vi "Convert TDMS to Excel.vi"(8 "error in":errorcluster, 9 "Show Configure Dialog?":bool, 10 "Remove Extra Properties? (T)":bool=TRUE, 11 "Path to TDMS/TDM File":path) -> (0 "error out":errorcluster)   [LabVIEW 2017]
doc: "This VI will convert a TDMS file to a XLSX file. Excel 2007, and the TDMS Add on for Excel needs to be installed. Then provide the path to the TDMS or TDM file. A file with the same name in the same directory will be created with a .XLSX file extension.\n\nBy default the conversion will remove many extra properties that aren't always used. To include all properties make \"Remove Extra Properties\" false. If you would like to choose the properties to include set \"Show Configure Dialog\" to be true.\n\nBrian Hoover (hooovahh) 2010"
uses:
  <userlib>/_OpenG.lib/file/file.llb/Strip Path Extension - String__ogtk.vi
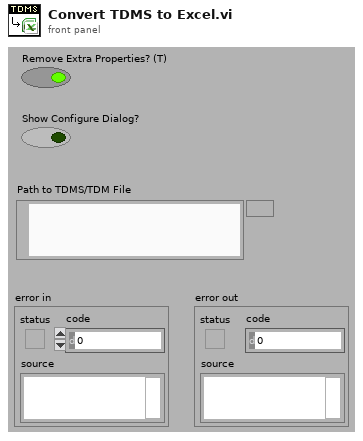
[diagram p1: front panel]
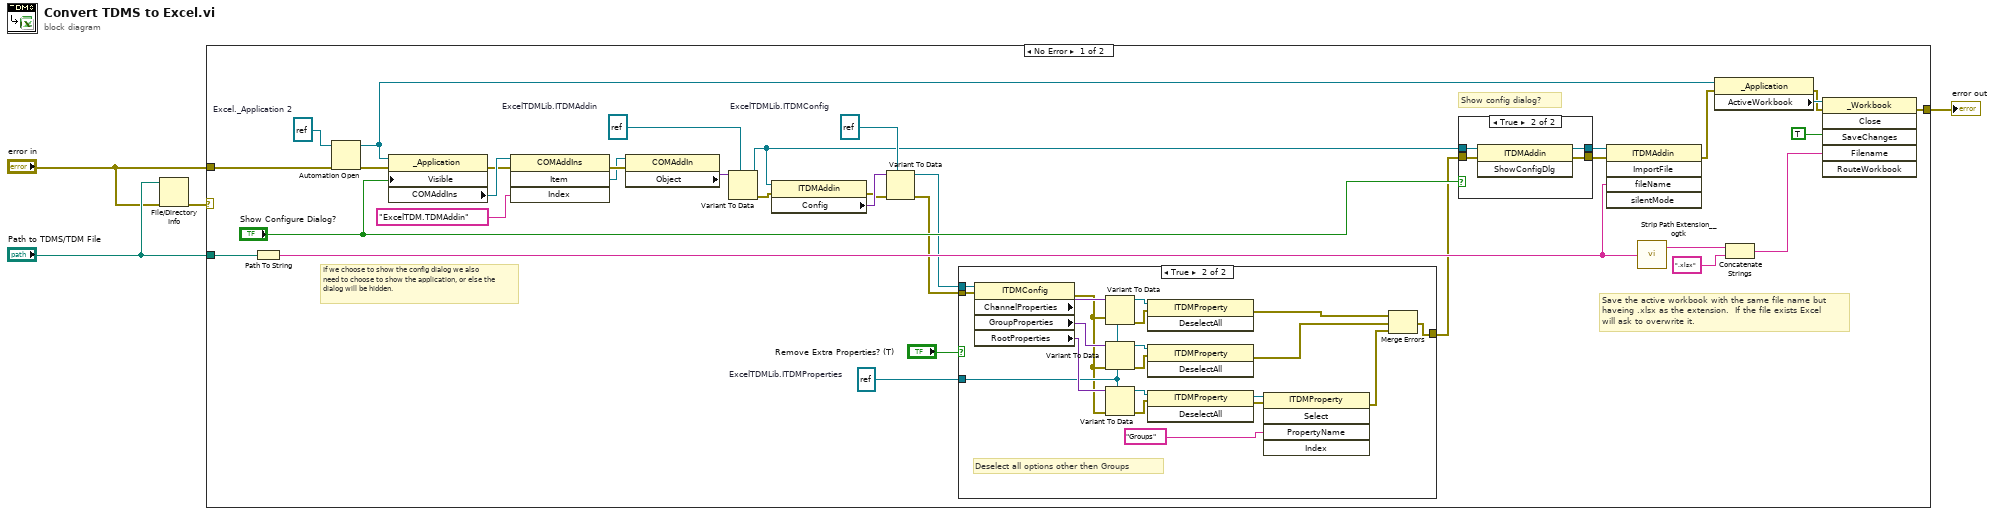
[diagram p0: block diagram]
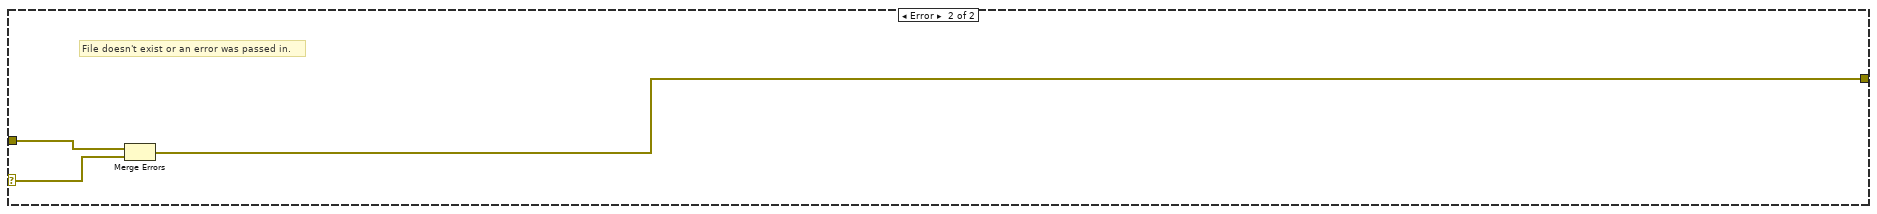
[diagram p4: hidden frame]
diagram:
  n1 = File/Directory Info(path="Path to TDMS/TDM File", error in="error in") -> (error out=w3:errorcluster)  [unwired: 6 out]
  n2 = case shown="No Error" w3 {
    selector: w3 -> [_ w67]
    tunnel: "Path to TDMS/TDM File" -> [w26 _]
    tunnel: [w21 w66] -> w1
    tunnel: "error in" -> [w19 w68]
    frame No Error {
      w36 = refnum<k7> refnum  # Excel._Application 2
      w13 = refnum<k7> refnum  # ExcelTDMLib.ITDMProperties
      w14 = refnum<k7> refnum  # ExcelTDMLib.ITDMConfig
      w37 = refnum<k7> refnum  # ExcelTDMLib.ITDMAddin
      # "Save the active workbook with the same file name but haveing .xlsx as the extension.  If the file exists Excel will ask to overwrite it."
      # "Show config dialog?"
      # "If we choose to show the config dialog we also need to choose to show the application, or else the dialog will be hidden."
      n3 = Path To String(path=w26) -> (string=w25:string)
      n4 = Automation Open(error in (no error)=w19, Automation Refnum=w36) -> (Automation Refnum=w30:refnum<k7>, error out=w35:errorcluster)  [unwired: 2 in]
      n5 = property class="_Application"(reference=w30, error in=w35, "Visible"="Show Configure Dialog?") -> (error out=w31:errorcluster, "COMAddIns"=w38:refnum<k7>)  [unwired: 1 out]
      n6 = invoke class="COMAddIns" method="Item"(reference=w38, error in=w31, "Index"="ExcelTDM.TDMAddin") -> (error out=w33:errorcluster, "Item"=w32:refnum<k7>)  [unwired: 1 in, 2 out]
      n7 = property class="COMAddIn"(reference=w32, error in=w33) -> ("Object"=w15:variant)  [unwired: 2 out]
      n8 = Variant To Data(type=w37, Variant=w15) -> (data=w12:refnum<k7>, error out=w10:errorcluster)  [unwired: 1 in]
      n9 = property class="ITDMAddin"(reference=w12, error in=w10) -> (error out=w9:errorcluster, "Config"=w11:variant)  [unwired: 1 out]
      n10 = Variant To Data(error in=w9, type=w14, Variant=w11) -> (data=w7:refnum<k7>, error out=w8:errorcluster)
      n11 = case shown="True" "Remove Extra Properties? (T)" {
        tunnel: w13 -> [_ w55]
        tunnel: w8 -> [w39 w46]
        tunnel: w7 -> [_ w45]
        tunnel: [w39 w44] -> w6
        frame False {
        }
        frame True {
          # "Deselect all options other then Groups"
          n12 = property class="ITDMConfig"(reference=w45, error in=w46) -> (error out=w50:errorcluster, "ChannelProperties"=w59:variant, "GroupProperties"=w57:variant, "RootProperties"=w56:variant)  [unwired: 1 out]
          n13 = Variant To Data(error in=w50, type=w55, Variant=w59) -> (data=w58:refnum<k7>, error out=w47:errorcluster)
          n14 = Variant To Data(error in=w50, type=w55, Variant=w57) -> (data=w53:refnum<k7>, error out=w48:errorcluster)
          n15 = Variant To Data(error in=w50, type=w55, Variant=w56) -> (data=w54:refnum<k7>, error out=w49:errorcluster)
          n16 = invoke class="ITDMProperty" method="DeselectAll"(reference=w58, error in=w47) -> (error out=w51:errorcluster)  [unwired: 1 in, 2 out]
          n17 = invoke class="ITDMProperty" method="DeselectAll"(reference=w53, error in=w48) -> (error out=w52:errorcluster)  [unwired: 1 in, 2 out]
          n18 = invoke class="ITDMProperty" method="DeselectAll"(reference=w54, error in=w49) -> (reference out=w43:refnum<k7>, error out=w42:errorcluster)  [unwired: 1 in, 1 out]
          n19 = invoke class="ITDMProperty" method="Select"(reference=w43, error in=w42, "PropertyName"="Groups" ("string")) -> (error out=w41:errorcluster)  [unwired: 2 in, 4 out]
          n20 = Merge Errors(w51, w52, w41) -> (w44:errorcluster)
        }
      }
      n21 = case shown="True" "Show Configure Dialog?" {
        tunnel: w12 -> [w61 w65]
        tunnel: w6 -> [w60 w64]
        tunnel: [w60 w63] -> w18
        tunnel: [w61 w62] -> w17
        frame False {
        }
        frame True {
          n22 = invoke class="ITDMAddin" method="ShowConfigDlg"(reference=w65, error in=w64) -> (reference out=w62:refnum<k7>, error out=w63:errorcluster)  [unwired: 1 in, 1 out]
        }
      }
      n23 = invoke class="ITDMAddin" method="ImportFile"(reference=w17, error in=w18, "fileName"=w25) -> (error out=w29:errorcluster)  [unwired: 2 in, 4 out]
      n24 = call-poly <userlib>:"Strip Path Extension__ogtk.vi"("path"=w25) -> ("root"=w24:string)  [unwired: 1 out]
      n25 = property class="_Application"(reference=w30, error in=w29) -> (error out=w20:errorcluster, "ActiveWorkbook"=w28:refnum<k7>)  [unwired: 1 out]
      n26 = Concatenate Strings(w24, ".xlsx" ("string")) -> (w22:string)
      n27 = invoke class="_Workbook" method="Close"(reference=w28, error in=w20, "SaveChanges"=TRUE, "Filename"=w22) -> (error out=w21:errorcluster)  [unwired: 2 in, 5 out]
    }
    frame Error {
      # "File doesn't exist or an error was passed in."
      n28 = Merge Errors(w68, w67) -> (w66:errorcluster)
    }
  }
  "error out" <- w1
